vi "Run.vi"(8 "error in (no error)":errorcluster, 11 "Channel in":refnum<class "ECHARPE_Channel.lvclass">) -> (0 "error out":errorcluster, 3 "Channel out":refnum<class "ECHARPE_Channel.lvclass">)   [LabVIEW 2018, in "ECHARPE_Channel.lvclass"]
doc: "Run the channel"
uses:
  ECHARPE_Channel.lvclass
  C:/Users/Denis/Desktop/S4ACS/S4ACS/Channel/Channel.lvclass
  Channel/Channel.lvclass/Channel.ctl
  Sim_CCD/Sim_CCD.lvclass
  State Machine/State Machine.lvclass
  RxTx/RxTx.lvclass
  Server/Server.lvclass
  Channel/Channel.lvclass
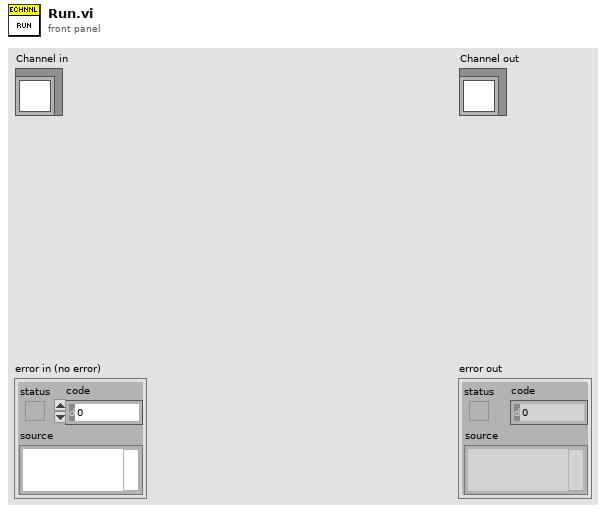
[diagram p1: front panel]
types:
  T1 = cluster{"State Machine.lvclass":refnum<class "State Machine.lvclass">, "RxTx.lvclass":refnum<class "RxTx.lvclass">, "Save_Header_RxTx.lvclass":refnum<class "RxTx.lvclass">, "Status SM.lvclass":refnum<class "State Machine.lvclass">, "Status RxTx.lvclass":refnum<class "RxTx.lvclass">, "servers array":refnum<class "Server.lvclass">[], "Events log file.lvclass":refnum<class "Log File.lvclass">, "Errors log file.lvclass":refnum<class "Log File.lvclass">, "Keywords log file.lvclass":refnum<class "Log File.lvclass">, "Sim_CCD.lvclass":refnum<class "Sim_CCD.lvclass">}
  T2 = cluster{"field 1":string, "field 2":string, "field 3":string}
  T3 = cluster{"PREAMP":u16, "READOUT_RATE":u16, "VERTICAL_SHIFT_SPEED":u16, "READ_MODE":u16, "VERTICAL_CLOCK_VOLTAGE":u16, "ACQUISITION_MODE":u16, "AD_CHANNEL":u16, "SHUTTER_TTL":u16, "SHUTTER_OPENING_TIME":u16, "SHUTTER_CLOSING_TIME":u16, "SHUTTER_MODE":u16, "TRIGGER_MODE":u16, "VBIN":u16, "INITIAL_LINE":u16, "INITIAL_COLUMN":u16, "FINAL_LINE":u16, "FINAL_COLUMN":u16, "HBIN":u16}
  T4 = typedef "LVDateTimeRec.ctl" = cluster{"fractional second":dbl, "second":i32, "minute":i32, "hour":i32, "day of month":i32, "month":i32, "year":i32, "day of week":i32, "day of year":i32, "DST":i32}
  T5 = cluster{"Time Acq Started":u32, "Image delay":u64, "Last update - CCD config":timestamp, "SYSTEMTIME":T4, "Readout time":dbl, "Time acq finished":u32, "effective exptime":dbl}
  T6 = cluster{"FRAMES_DONE":u16, "CCD_STATUS":string, "CURRENT_TEMPERATURE":i16, "TEMPERATURE_STATUS":string, "FRAME_EXPOSURE_TIME":dbl, "SERIAL_NUMBER":u16, "ACQUIRING":bool, "POWER":bool, "ACS MODE":bool}
  T7 = cluster{"Stop Acquisition":bool, "Abort Acquisition":bool, "Pause acquisition":bool, "wait expose command":bool, "video mode":bool, "stop app":bool}
  T8 = cluster{"CYCLES_DONE":u16, "LAST_IMAGE_NAME":string, "USED_DISK_SPACE":u16, "IMAGE_INDEX":u32, "acquisition error":bool}
  T9 = cluster{"EXPTIME":dbl, "#FRAMES":u32, "COOLER_POWER_STATUS":u16, "TEMP":i32}
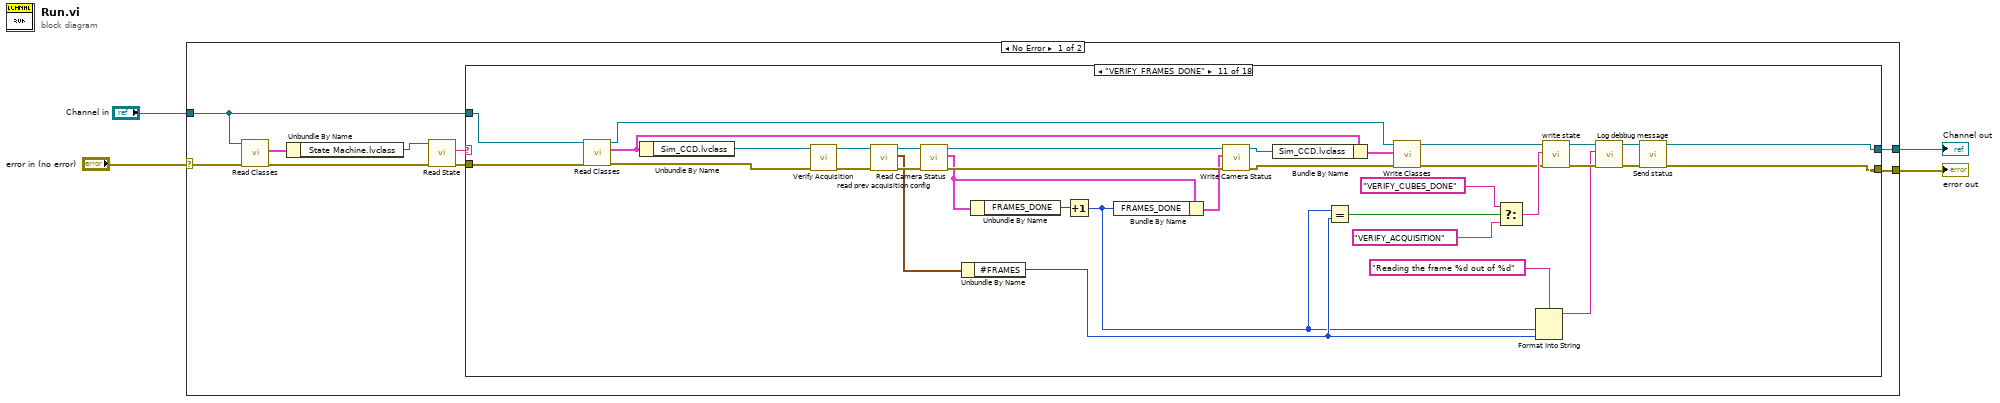
[diagram p0: block diagram]
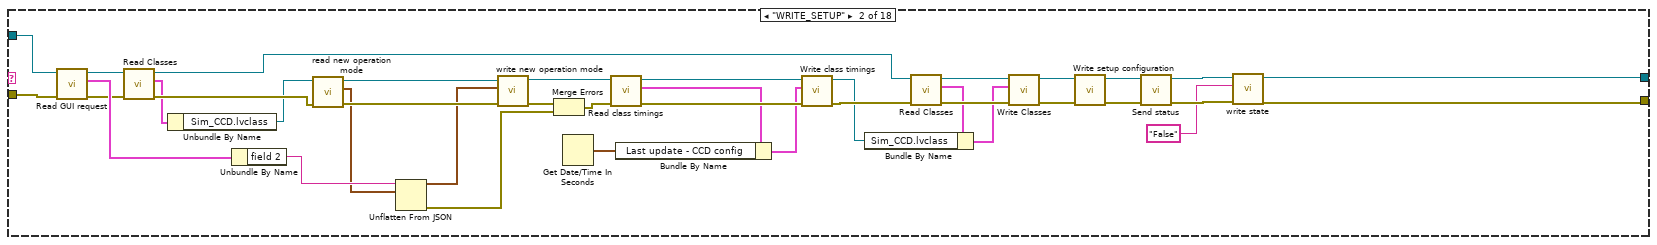
[diagram p3: hidden frame]
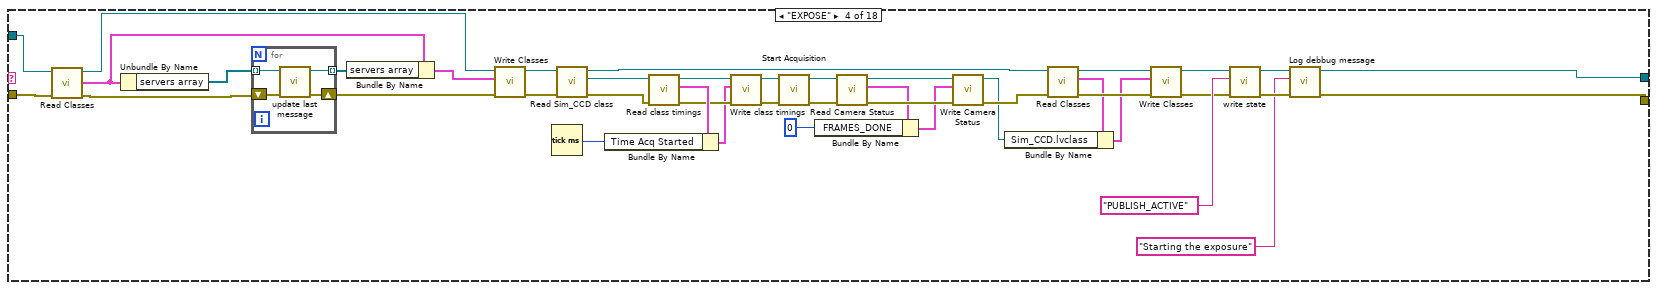
[diagram p5: hidden frame]
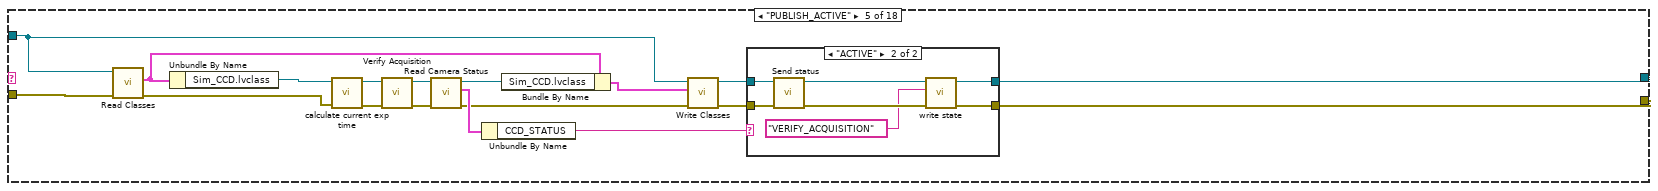
[diagram p6: hidden frame]
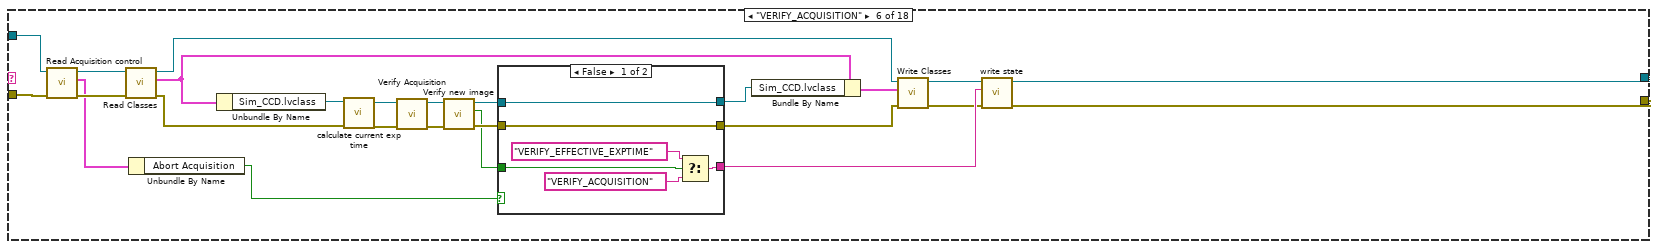
[diagram p8: hidden frame]
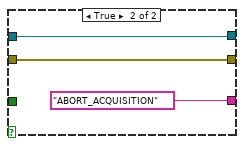
[diagram p9: hidden frame]
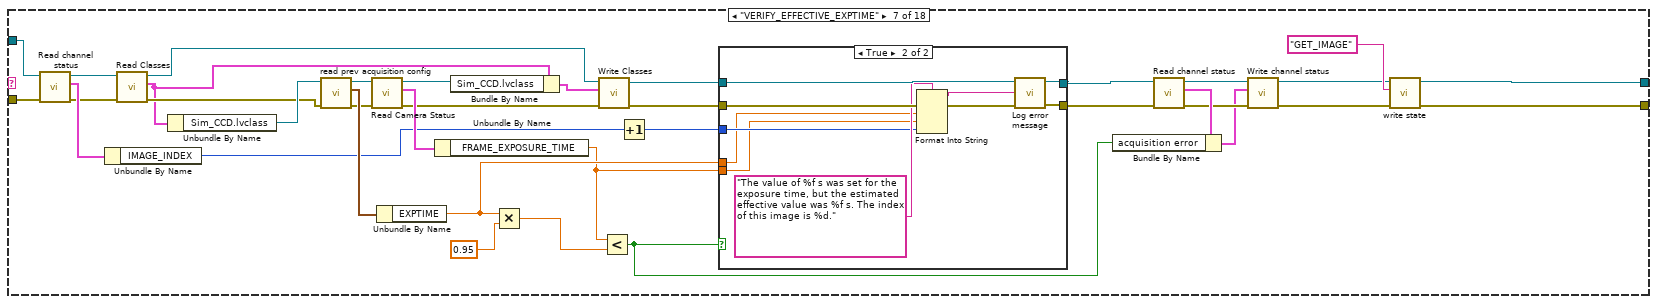
[diagram p10: hidden frame]
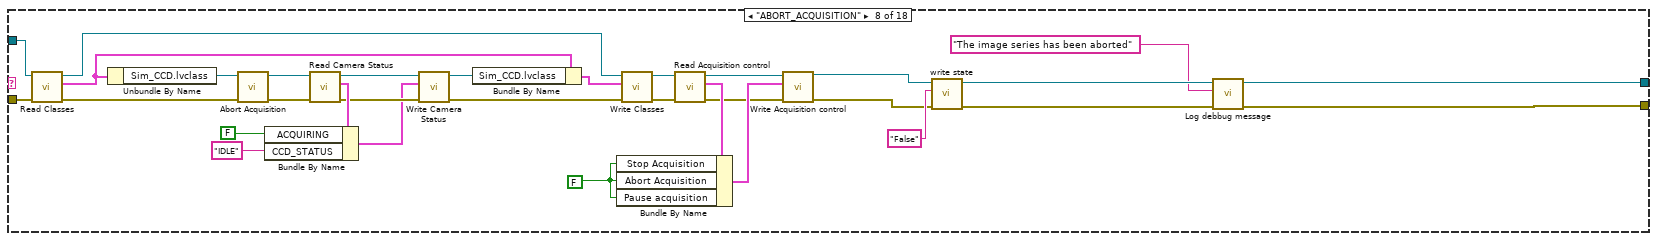
[diagram p12: hidden frame]
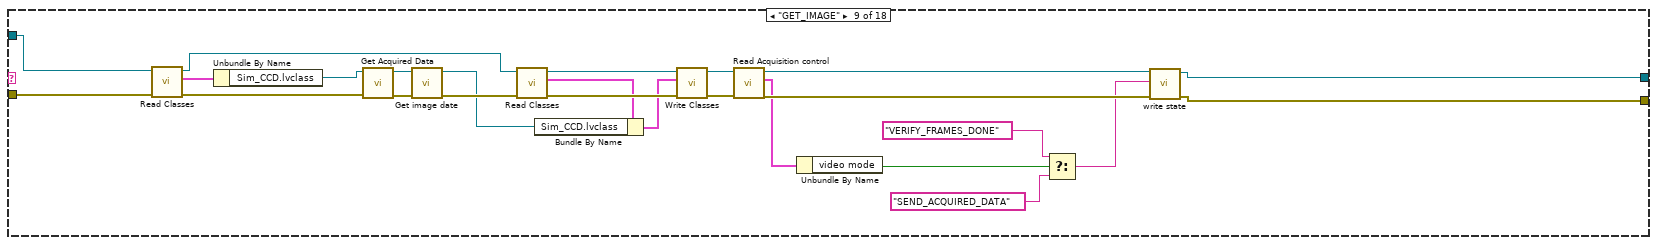
[diagram p13: hidden frame]
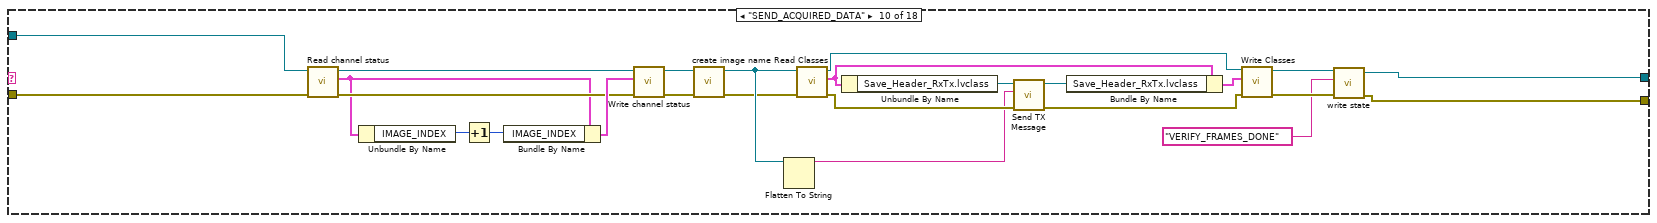
[diagram p14: hidden frame]
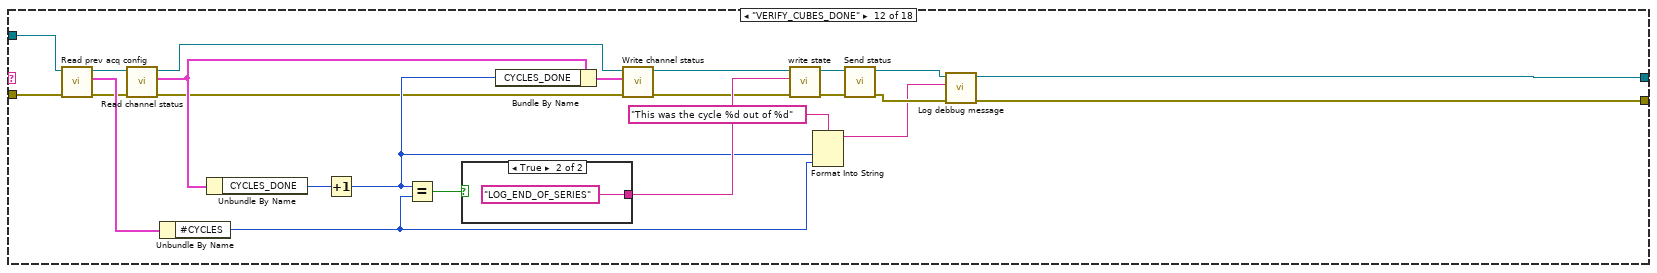
[diagram p15: hidden frame]
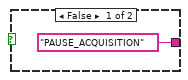
[diagram p16: hidden frame]
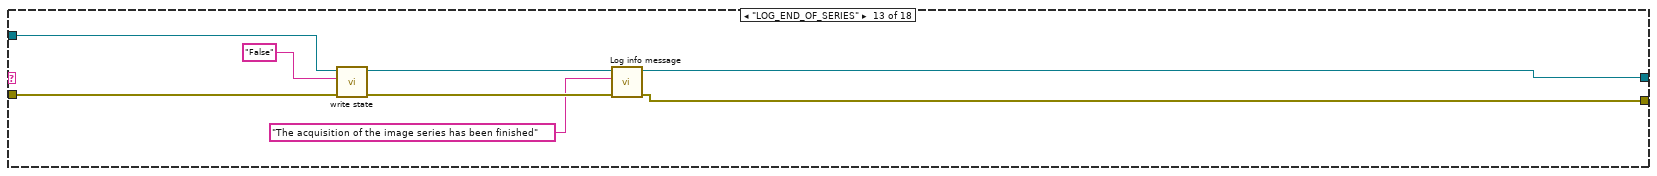
[diagram p17: hidden frame]
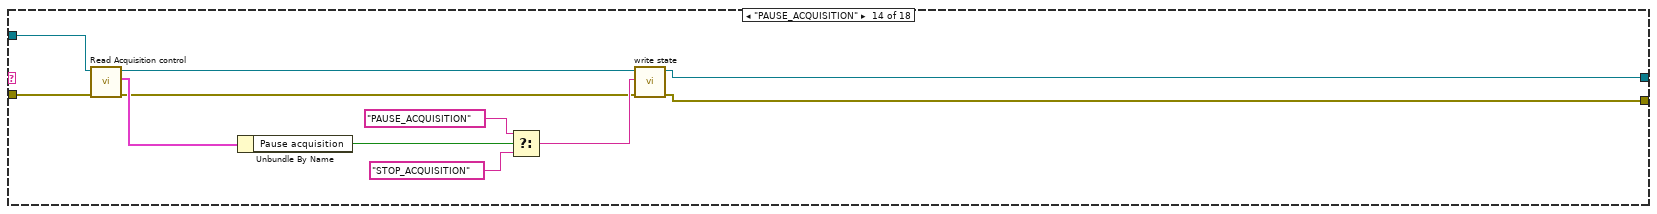
[diagram p18: hidden frame]
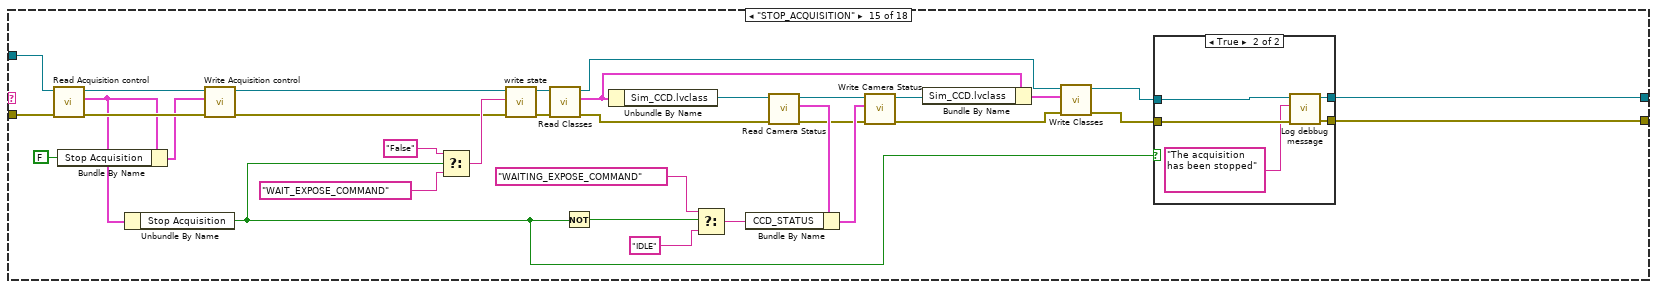
[diagram p19: hidden frame]
diagram:
  n1 = case shown="No Error" "error in (no error)" {
    selector: "error in (no error)" -> [w7 w552]
    tunnel: [w13 w552] -> w3
    tunnel: [w12 w551] -> w1
    tunnel: "Channel in" -> [w8 w551]
    frame No Error {
      n2 = call-dynamic "Read Classes.vi"("error in (no error)"=w7, "Channel in"=w8) -> ("error out"=w6:errorcluster, "Classes"=w9:T1)  [unwired: 7 in, 1 out]
      n3 = Unbundle By Name(w9) -> ("State Machine.lvclass"=w5:refnum<class "State Machine.lvclass">)
      n4 = call-dynamic "Read State.vi"("error in (no error)"=w6, "State Machine in"=w5) -> ("error out"=w11:errorcluster, "State"=w10:string)  [unwired: 7 in, 1 out]
      n5 = case shown="\"VERIFY_FRAMES_DONE\"" w10 {
        tunnel: w11 -> [w14 w36 w54 w77 w111 w134 w175 w228 w262 w271 w317 w334 w360 w364 w391 w416 w425 w432]
        tunnel: [w14 w23 w54 w87 w118 w150 w197 w231 w253 w291 w316 w346 w356 w370 w394 w422 w425 w442] -> w13
        tunnel: [w15 w24 w55 w88 w119 w151 w198 w232 w252 w292 w315 w345 w357 w369 w395 w421 w426 w443] -> w12
        tunnel: w8 -> [w15 w38 w55 w76 w106 w132 w169 w227 w263 w272 w318 w332 w361 w365 w392 w417 w426 w431]
        frame "False", Default {
        }
        frame "WRITE_SETUP" {
          n6 = call "Read GUI request.vi"("error in (no error)"=w36, "Channel in"=w38) -> ("error out"=w37:errorcluster, "GUI request"=w42:T2, "Channel out"=w39:refnum<class "ECHARPE_Channel.lvclass">)  [unwired: 7 in]
          n7 = call-dynamic "Read Classes.vi"("error in (no error)"=w37, "Channel in"=w39) -> ("error out"=w40:errorcluster, "Classes"=w17:T1, "Channel out"=w29:refnum<class "ECHARPE_Channel.lvclass">)  [unwired: 7 in]
          n8 = Unbundle By Name(w17) -> ("Sim_CCD.lvclass"=w16:refnum<class "Sim_CCD.lvclass">)
          n9 = Unbundle By Name(w42) -> ("field 2"=w41:string)
          n10 = call "read new operation mode.vi"("error in (no error)"=w40, "CCDCamera in"=w16) -> ("error out"=w52:errorcluster, "new operation mode"=w19:T3, "CCDCamera out"=w53:refnum<class "Sim_CCD.lvclass">)  [unwired: 7 in]
          n11 = Unflatten From JSON(JSON string=w41, type and defaults=w19) -> (value=w18:T3, error out=w43:errorcluster)  [unwired: 5 in]
          n12 = call "write new operation mode.vi"("error in (no error)"=w52, "new operation mode"=w18, "CCDCamera in"=w53) -> ("error out"=w45:errorcluster, "CCDCamera out"=w51:refnum<class "Sim_CCD.lvclass">)  [unwired: 7 in]
          n13 = Merge Errors(w45, w43) -> (w44:errorcluster)
          n14 = Get Date/Time In Seconds() -> (seconds since 1Jan1904=w46:timestamp)
          n15 = call "Read class timings.vi"("error in (no error)"=w44, "Simulated Camera in"=w51) -> ("error out"=w49:errorcluster, "class timings"=w48:T5, "Simulated Camera out"=w50:refnum<class "Sim_CCD.lvclass">)  [unwired: 7 in]
          n16 = Bundle By Name(cluster=w48, "Last update - CCD config"=w46) -> (w47:T5)
          n17 = call "Write class timings.vi"("error in (no error)"=w49, "class timings"=w47, "Simulated Camera in"=w50) -> ("error out"=w33:errorcluster, "Simulated Camera out"=w31:refnum<class "Sim_CCD.lvclass">)  [unwired: 7 in]
          n18 = call-dynamic "Read Classes.vi"("error in (no error)"=w33, "Channel in"=w29) -> ("error out"=w34:errorcluster, "Classes"=w32:T1, "Channel out"=w35:refnum<class "ECHARPE_Channel.lvclass">)  [unwired: 7 in]
          n19 = Bundle By Name(cluster=w32, "Sim_CCD.lvclass"=w31) -> (w30:T1)
          n20 = call-dynamic "Write Classes.vi"("error in (no error)"=w34, "Classes"=w30, "Channel in"=w35) -> ("error out"=w25:errorcluster, "Channel out"=w27:refnum<class "ECHARPE_Channel.lvclass">)  [unwired: 7 in]
          n21 = call "Write setup configuration.vi"("error in (no error)"=w25, "Channel in"=w27) -> ("error out"=w26:errorcluster, "Channel out"=w28:refnum<class "ECHARPE_Channel.lvclass">)  [unwired: 8 in]
          n22 = call-dynamic "Send status.vi"("error in (no error)"=w26, "Channel in"=w28) -> ("error out"=w21:errorcluster, "Channel out"=w22:refnum<class "ECHARPE_Channel.lvclass">)  [unwired: 8 in]
          n23 = call "write state.vi"("error in (no error)"=w21, "state"="False", "Channel in"=w22) -> ("error out"=w23:errorcluster, "Channel out"=w24:refnum<class "ECHARPE_Channel.lvclass">)  [unwired: 7 in]
        }
        frame "---------------------------------" {
        }
        frame "EXPOSE" {
          n24 = call-dynamic "Read Classes.vi"("error in (no error)"=w77, "Channel in"=w76) -> ("error out"=w73:errorcluster, "Classes"=w70:T1, "Channel out"=w74:refnum<class "ECHARPE_Channel.lvclass">)  [unwired: 7 in]
          n25 = Unbundle By Name(w70) -> ("servers array"=w75:refnum<class "Server.lvclass">[])
          n26 = for {
            tunnel: w75 -> [w98] mode=indexing
            shift-right: [w101] -> w72
            shift-left: w73 -> [w99]
            tunnel: [w100] -> w69 mode=indexing
            n27 = call "update last message.vi"("error in (no error)"=w99, "Server in"=w98) -> ("error out"=w101:errorcluster, "Server out"=w100:refnum<class "Server.lvclass">)  [unwired: 8 in]
          }
          n28 = Bundle By Name(cluster=w70, "servers array"=w69) -> (w71:T1)
          n29 = call-dynamic "Write Classes.vi"("error in (no error)"=w72, "Classes"=w71, "Channel in"=w74) -> ("error out"=w66:errorcluster, "Channel out"=w67:refnum<class "ECHARPE_Channel.lvclass">)  [unwired: 7 in]
          n30 = Tick Count (ms)() -> (millisecond timer value=w78:u32)
          n31 = call "Read Sim_CCD class.vi"("error in (no error)"=w66, "Channel in"=w67) -> ("error out"=w65:errorcluster, "Sim_CCD.lvclass"=w68:refnum<class "Sim_CCD.lvclass">, "Channel out"=w59:refnum<class "ECHARPE_Channel.lvclass">)  [unwired: 7 in]
          n32 = call "Read class timings.vi"("error in (no error)"=w65, "Simulated Camera in"=w68) -> ("error out"=w81:errorcluster, "class timings"=w82:T5, "Simulated Camera out"=w80:refnum<class "Sim_CCD.lvclass">)  [unwired: 7 in]
          n33 = Bundle By Name(cluster=w82, "Time Acq Started"=w78) -> (w79:T5)
          n34 = call "Write class timings.vi"("error in (no error)"=w81, "class timings"=w79, "Simulated Camera in"=w80) -> ("error out"=w84:errorcluster, "Simulated Camera out"=w83:refnum<class "Sim_CCD.lvclass">)  [unwired: 7 in]
          n35 = call-dynamic "Start Acquisition.vi"("error in (no error)"=w84, "CCDCamera in"=w83) -> ("error out"=w90:errorcluster, "CCDCamera out"=w91:refnum<class "Sim_CCD.lvclass">)  [unwired: 8 in]
          n36 = call "Read Camera Status.vi"("error in (no error)"=w90, "CCDCamera in"=w91) -> ("error out"=w97:errorcluster, "camera status"=w95:T6, "CCDCamera out"=w96:refnum<class "Sim_CCD.lvclass">)  [unwired: 7 in]
          n37 = Bundle By Name(cluster=w95, "FRAMES_DONE"=u16 0) -> (w94:T6)
          n38 = call "Write Camera Status.vi"("error in (no error)"=w97, "camera status"=w94, "CCDCamera in"=w96) -> ("error out"=w64:errorcluster, "CCDCamera out"=w56:refnum<class "Sim_CCD.lvclass">)  [unwired: 7 in]
          n39 = call-dynamic "Read Classes.vi"("error in (no error)"=w64, "Channel in"=w59) -> ("error out"=w61:errorcluster, "Classes"=w58:T1, "Channel out"=w60:refnum<class "ECHARPE_Channel.lvclass">)  [unwired: 7 in]
          n40 = Bundle By Name(cluster=w58, "Sim_CCD.lvclass"=w56) -> (w57:T1)
          n41 = call-dynamic "Write Classes.vi"("error in (no error)"=w61, "Classes"=w57, "Channel in"=w60) -> ("error out"=w63:errorcluster, "Channel out"=w62:refnum<class "ECHARPE_Channel.lvclass">)  [unwired: 7 in]
          n42 = call "write state.vi"("error in (no error)"=w63, "state"="PUBLISH_ACTIVE", "Channel in"=w62) -> ("error out"=w86:errorcluster, "Channel out"=w89:refnum<class "ECHARPE_Channel.lvclass">)  [unwired: 7 in]
          n43 = call "Log debbug message.vi"("error in (no error)"=w86, "String"="Starting the exposure", "Channel in"=w89) -> ("error out"=w87:errorcluster, "Channel out"=w88:refnum<class "ECHARPE_Channel.lvclass">)  [unwired: 7 in]
        }
        frame "PUBLISH_ACTIVE" {
          n44 = call-dynamic "Read Classes.vi"("error in (no error)"=w111, "Channel in"=w106) -> ("error out"=w109:errorcluster, "Classes"=w104:T1)  [unwired: 7 in, 1 out]
          n45 = Unbundle By Name(w104) -> ("Sim_CCD.lvclass"=w110:refnum<class "Sim_CCD.lvclass">)
          n46 = call-dynamic "calculate current exp time.vi"("error in (no error)"=w109, "CCDCamera in"=w110) -> ("error out"=w112:errorcluster, "CCDCamera out"=w113:refnum<class "Sim_CCD.lvclass">)  [unwired: 8 in]
          n47 = call-dynamic "Verify Acquisition.vi"("error in (no error)"=w112, "CCDCamera in"=w113) -> ("error out"=w114:errorcluster, "CCDCamera out"=w115:refnum<class "Sim_CCD.lvclass">)  [unwired: 8 in]
          n48 = call "Read Camera Status.vi"("error in (no error)"=w114, "CCDCamera in"=w115) -> ("error out"=w105:errorcluster, "camera status"=w117:T6, "CCDCamera out"=w103:refnum<class "Sim_CCD.lvclass">)  [unwired: 7 in]
          n49 = Unbundle By Name(w117) -> ("CCD_STATUS"=w116:string)
          n50 = Bundle By Name(cluster=w104, "Sim_CCD.lvclass"=w103) -> (w102:T1)
          n51 = call-dynamic "Write Classes.vi"("error in (no error)"=w105, "Classes"=w102, "Channel in"=w106) -> ("error out"=w107:errorcluster, "Channel out"=w108:refnum<class "ECHARPE_Channel.lvclass">)  [unwired: 7 in]
          n52 = case shown="\"ACTIVE\"" w116 {
            tunnel: w108 -> [w121 w124]
            tunnel: [w121 w128] -> w119
            tunnel: [w120 w127] -> w118
            tunnel: w107 -> [w120 w123]
            frame "False", Default {
            }
            frame "ACTIVE" {
              n53 = call-dynamic "Send status.vi"("error in (no error)"=w123, "Channel in"=w124) -> ("error out"=w126:errorcluster, "Channel out"=w125:refnum<class "ECHARPE_Channel.lvclass">)  [unwired: 8 in]
              n54 = call "write state.vi"("error in (no error)"=w126, "state"="VERIFY_ACQUISITION", "Channel in"=w125) -> ("error out"=w127:errorcluster, "Channel out"=w128:refnum<class "ECHARPE_Channel.lvclass">)  [unwired: 7 in]
            }
          }
        }
        frame "VERIFY_ACQUISITION" {
          n55 = call "Read Acquisition control.vi"("error in (no error)"=w134, "Channel in"=w132) -> ("error out"=w133:errorcluster, "Acquisition control"=w130:T7, "Channel out"=w131:refnum<class "ECHARPE_Channel.lvclass">)  [unwired: 7 in]
          n56 = call-dynamic "Read Classes.vi"("error in (no error)"=w133, "Channel in"=w131) -> ("error out"=w140:errorcluster, "Classes"=w137:T1, "Channel out"=w139:refnum<class "ECHARPE_Channel.lvclass">)  [unwired: 7 in]
          n57 = Unbundle By Name(w130) -> ("Abort Acquisition"=w129:bool)
          n58 = Unbundle By Name(w137) -> ("Sim_CCD.lvclass"=w138:refnum<class "Sim_CCD.lvclass">)
          n59 = call-dynamic "calculate current exp time.vi"("error in (no error)"=w140, "CCDCamera in"=w138) -> ("error out"=w146:errorcluster, "CCDCamera out"=w147:refnum<class "Sim_CCD.lvclass">)  [unwired: 8 in]
          n60 = call-dynamic "Verify Acquisition.vi"("error in (no error)"=w146, "CCDCamera in"=w147) -> ("error out"=w153:errorcluster, "CCDCamera out"=w152:refnum<class "Sim_CCD.lvclass">)  [unwired: 8 in]
          n61 = call-dynamic "Verify new image.vi"("error in (no error)"=w153, "CCDCamera in"=w152) -> ("error out"=w148:errorcluster, "New Images ?"=w144:bool, "CCDCamera out"=w149:refnum<class "Sim_CCD.lvclass">)  [unwired: 7 in]
          n62 = case shown="False" w129 {
            tunnel: w149 -> [w159 w162]
            tunnel: w148 -> [w158 w161]
            tunnel: [w159 w162] -> w135
            tunnel: [w158 w161] -> w141
            tunnel: [w155 "ABORT_ACQUISITION"] -> w145
            tunnel: w144 -> [w154 _]
            frame False {
              n63 = Select(t="VERIFY_EFFECTIVE_EXPTIME", s=w154, f="VERIFY_ACQUISITION") -> (s? t:f=w155:string)
            }
            frame True {
            }
          }
          n64 = Bundle By Name(cluster=w137, "Sim_CCD.lvclass"=w135) -> (w136:T1)
          n65 = call-dynamic "Write Classes.vi"("error in (no error)"=w141, "Classes"=w136, "Channel in"=w139) -> ("error out"=w143:errorcluster, "Channel out"=w142:refnum<class "ECHARPE_Channel.lvclass">)  [unwired: 7 in]
          n66 = call "write state.vi"("error in (no error)"=w143, "state"=w145, "Channel in"=w142) -> ("error out"=w150:errorcluster, "Channel out"=w151:refnum<class "ECHARPE_Channel.lvclass">)  [unwired: 7 in]
        }
        frame "VERIFY_EFFECTIVE_EXPTIME" {
          n67 = call-dynamic "Read channel status.vi"("error in (no error)"=w175, "Channel in"=w169) -> ("error out"=w174:errorcluster, "channel status"=w177:T8, "Channel out"=w173:refnum<class "ECHARPE_Channel.lvclass">)  [unwired: 7 in]
          n68 = Unbundle By Name(w177) -> ("IMAGE_INDEX"=w176:u32)
          n69 = call-dynamic "Read Classes.vi"("error in (no error)"=w174, "Channel in"=w173) -> ("error out"=w171:errorcluster, "Classes"=w165:T1, "Channel out"=w168:refnum<class "ECHARPE_Channel.lvclass">)  [unwired: 7 in]
          n70 = Unbundle By Name(w165) -> ("Sim_CCD.lvclass"=w172:refnum<class "Sim_CCD.lvclass">)
          n71 = call "read prev acquisition config.vi"("error in (no error)"=w171, "Simulated_CCD_Camera in"=w172) -> ("error out"=w191:errorcluster, "prev acquisition configuration"=w193:T9, "Simulated_CCD_Camera out"=w192:refnum<class "Sim_CCD.lvclass">)  [unwired: 7 in]
          n72 = call "Read Camera Status.vi"("error in (no error)"=w191, "CCDCamera in"=w192) -> ("error out"=w166:errorcluster, "camera status"=w190:T6, "CCDCamera out"=w163:refnum<class "Sim_CCD.lvclass">)  [unwired: 7 in]
          n73 = Unbundle By Name(w193) -> ("EXPTIME"=w188:dbl)
          n74 = Unbundle By Name(w190) -> ("FRAME_EXPOSURE_TIME"=w187:dbl)
          n75 = Bundle By Name(cluster=w165, "Sim_CCD.lvclass"=w163) -> (w164:T1)
          n76 = Multiply(x=w188, y=0.95) -> (x*y=w194:dbl)
          n77 = call-dynamic "Write Classes.vi"("error in (no error)"=w166, "Classes"=w164, "Channel in"=w168) -> ("error out"=w170:errorcluster, "Channel out"=w167:refnum<class "ECHARPE_Channel.lvclass">)  [unwired: 7 in]
          n78 = Less?(x=w187, y=w194) -> (x < y?=w185:bool)
          n79 = Increment(x=w176) -> (x+1=w189:u32)
          n80 = case shown="True" w185 {
            tunnel: w167 -> [w200 w210]
            tunnel: [w200 w209] -> w184
            tunnel: [w199 w208] -> w183
            tunnel: w170 -> [w199 w207]
            tunnel: w189 -> [_ w203]
            tunnel: w188 -> [_ w202]
            tunnel: w187 -> [_ w201]
            frame False {
            }
            frame True {
              n81 = Format Into String(format string="The value of %f s was set for the exposure time, but the estimated effective value was %f s. The index of this image is %d.", error in=w207, w202, w201, w203) -> (resulting string=w204:string, error out=w206:errorcluster)  [unwired: 1 in]
              n82 = call "Log error message.vi"("error in (no error)"=w206, "String"=w204, "Channel in"=w210) -> ("error out"=w208:errorcluster, "Channel out"=w209:refnum<class "ECHARPE_Channel.lvclass">)  [unwired: 7 in]
            }
          }
          n83 = call-dynamic "Read channel status.vi"("error in (no error)"=w183, "Channel in"=w184) -> ("error out"=w179:errorcluster, "channel status"=w186:T8, "Channel out"=w180:refnum<class "ECHARPE_Channel.lvclass">)  [unwired: 7 in]
          n84 = Bundle By Name(cluster=w186, "acquisition error"=w185) -> (w178:T8)
          n85 = call-dynamic "Write channel status.vi"("error in (no error)"=w179, "channel status"=w178, "Channel in"=w180) -> ("error out"=w182:errorcluster, "Channel out"=w181:refnum<class "ECHARPE_Channel.lvclass">)  [unwired: 7 in]
          n86 = call "write state.vi"("error in (no error)"=w182, "state"="GET_IMAGE", "Channel in"=w181) -> ("error out"=w197:errorcluster, "Channel out"=w198:refnum<class "ECHARPE_Channel.lvclass">)  [unwired: 7 in]
        }
        frame "ABORT_ACQUISITION" {
          w211 = FALSE ("Acquiring")
          n87 = call-dynamic "Read Classes.vi"("error in (no error)"=w228, "Channel in"=w227) -> ("error out"=w225:errorcluster, "Classes"=w221:T1, "Channel out"=w220:refnum<class "ECHARPE_Channel.lvclass">)  [unwired: 7 in]
          n88 = Unbundle By Name(w221) -> ("Sim_CCD.lvclass"=w226:refnum<class "Sim_CCD.lvclass">)
          n89 = call-dynamic "Abort Acquisition.vi"("error in (no error)"=w225, "CCDCamera in"=w226) -> ("error out"=w239:errorcluster, "CCDCamera out"=w240:refnum<class "Sim_CCD.lvclass">)  [unwired: 8 in]
          n90 = call "Read Camera Status.vi"("error in (no error)"=w239, "CCDCamera in"=w240) -> ("error out"=w237:errorcluster, "camera status"=w242:T6, "CCDCamera out"=w238:refnum<class "Sim_CCD.lvclass">)  [unwired: 7 in]
          n91 = Bundle By Name(cluster=w242, "ACQUIRING"=FALSE ("Acquiring"), "CCD_STATUS"="IDLE" ("STATUS")) -> (w236:T6)
          n92 = call "Write Camera Status.vi"("error in (no error)"=w237, "camera status"=w236, "CCDCamera in"=w238) -> ("error out"=w223:errorcluster, "CCDCamera out"=w224:refnum<class "Sim_CCD.lvclass">)  [unwired: 7 in]
          n93 = Bundle By Name(cluster=w221, "Sim_CCD.lvclass"=w224) -> (w222:T1)
          n94 = call-dynamic "Write Classes.vi"("error in (no error)"=w223, "Classes"=w222, "Channel in"=w220) -> ("error out"=w218:errorcluster, "Channel out"=w219:refnum<class "ECHARPE_Channel.lvclass">)  [unwired: 7 in]
          n95 = call "Read Acquisition control.vi"("error in (no error)"=w218, "Channel in"=w219) -> ("error out"=w212:errorcluster, "Acquisition control"=w214:T7, "Channel out"=w217:refnum<class "ECHARPE_Channel.lvclass">)  [unwired: 7 in]
          n96 = Bundle By Name(cluster=w214, "Stop Acquisition"=w211, "Abort Acquisition"=w211, "Pause acquisition"=w211) -> (w213:T7)
          n97 = call "Write Acquisition control.vi"("error in (no error)"=w212, "Acquisition control"=w213, "Channel in"=w217) -> ("error out"=w215:errorcluster, "Channel out"=w216:refnum<class "ECHARPE_Channel.lvclass">)  [unwired: 7 in]
          n98 = call "write state.vi"("error in (no error)"=w215, "state"="False", "Channel in"=w216) -> ("error out"=w230:errorcluster, "Channel out"=w233:refnum<class "ECHARPE_Channel.lvclass">)  [unwired: 7 in]
          n99 = call "Log debbug message.vi"("error in (no error)"=w230, "String"="The image series has been aborted", "Channel in"=w233) -> ("error out"=w231:errorcluster, "Channel out"=w232:refnum<class "ECHARPE_Channel.lvclass">)  [unwired: 7 in]
        }
        frame "GET_IMAGE" {
          n100 = call-dynamic "Read Classes.vi"("error in (no error)"=w262, "Channel in"=w263) -> ("error out"=w260:errorcluster, "Classes"=w261:T1, "Channel out"=w258:refnum<class "ECHARPE_Channel.lvclass">)  [unwired: 7 in]
          n101 = Unbundle By Name(w261) -> ("Sim_CCD.lvclass"=w259:refnum<class "Sim_CCD.lvclass">)
          n102 = call-dynamic "Get Acquired Data.vi"("error in (no error)"=w260, "CCDCamera in"=w259) -> ("error out"=w266:errorcluster, "CCDCamera out"=w267:refnum<class "Sim_CCD.lvclass">)  [unwired: 8 in]
          n103 = call-dynamic "Get image date.vi"("error in (no error)"=w266, "Simulated_CCD_Camera in"=w267) -> ("error out"=w265:errorcluster, "Simulated_CCD_Camera out"=w264:refnum<class "Sim_CCD.lvclass">)  [unwired: 8 in]
          n104 = call-dynamic "Read Classes.vi"("error in (no error)"=w265, "Channel in"=w258) -> ("error out"=w257:errorcluster, "Classes"=w256:T1, "Channel out"=w255:refnum<class "ECHARPE_Channel.lvclass">)  [unwired: 7 in]
          n105 = Bundle By Name(cluster=w256, "Sim_CCD.lvclass"=w264) -> (w254:T1)
          n106 = call-dynamic "Write Classes.vi"("error in (no error)"=w257, "Classes"=w254, "Channel in"=w255) -> ("error out"=w250:errorcluster, "Channel out"=w251:refnum<class "ECHARPE_Channel.lvclass">)  [unwired: 7 in]
          n107 = call "Read Acquisition control.vi"("error in (no error)"=w250, "Channel in"=w251) -> ("error out"=w248:errorcluster, "Acquisition control"=w247:T7, "Channel out"=w249:refnum<class "ECHARPE_Channel.lvclass">)  [unwired: 7 in]
          n108 = Unbundle By Name(w247) -> ("video mode"=w246:bool)
          n109 = Select(t="VERIFY_FRAMES_DONE", s=w246, f="SEND_ACQUIRED_DATA") -> (s? t:f=w243:string)
          n110 = call "write state.vi"("error in (no error)"=w248, "state"=w243, "Channel in"=w249) -> ("error out"=w253:errorcluster, "Channel out"=w252:refnum<class "ECHARPE_Channel.lvclass">)  [unwired: 7 in]
        }
        frame "SEND_ACQUIRED_DATA" {
          n111 = call-dynamic "Read channel status.vi"("error in (no error)"=w271, "Channel in"=w272) -> ("error out"=w278:errorcluster, "channel status"=w270:T8, "Channel out"=w277:refnum<class "ECHARPE_Channel.lvclass">)  [unwired: 7 in]
          n112 = Unbundle By Name(w270) -> ("IMAGE_INDEX"=w269:u32)
          n113 = Increment(x=w269) -> (x+1=w268:u32)
          n114 = Bundle By Name(cluster=w270, "IMAGE_INDEX"=w268) -> (w279:T8)
          n115 = call-dynamic "Write channel status.vi"("error in (no error)"=w278, "channel status"=w279, "Channel in"=w277) -> ("error out"=w273:errorcluster, "Channel out"=w274:refnum<class "ECHARPE_Channel.lvclass">)  [unwired: 7 in]
          n116 = call-dynamic "create image name.vi"("error in (no error)"=w273, "Channel in"=w274) -> ("error out"=w275:errorcluster, "Channel out"=w276:refnum<class "ECHARPE_Channel.lvclass">)  [unwired: 8 in]
          n117 = Flatten To String(anything=w276) -> (data string=w281:string)  [unwired: 3 in, 2 out]
          n118 = call-dynamic "Read Classes.vi"("error in (no error)"=w275, "Channel in"=w276) -> ("error out"=w286:errorcluster, "Classes"=w285:T1, "Channel out"=w280:refnum<class "ECHARPE_Channel.lvclass">)  [unwired: 7 in]
          n119 = Unbundle By Name(w285) -> ("Save_Header_RxTx.lvclass"=w287:refnum<class "RxTx.lvclass">)
          n120 = call "Send TX Message.vi"("error in (no error)"=w286, "message"=w281, "RxTx in"=w287) -> ("error out"=w282:errorcluster, "RxTx out"=w283:refnum<class "RxTx.lvclass">)  [unwired: 7 in]
          n121 = Bundle By Name(cluster=w285, "Save_Header_RxTx.lvclass"=w283) -> (w284:T1)
          n122 = call-dynamic "Write Classes.vi"("error in (no error)"=w282, "Classes"=w284, "Channel in"=w280) -> ("error out"=w290:errorcluster, "Channel out"=w289:refnum<class "ECHARPE_Channel.lvclass">)  [unwired: 7 in]
          n123 = call "write state.vi"("error in (no error)"=w290, "state"="VERIFY_FRAMES_DONE", "Channel in"=w289) -> ("error out"=w291:errorcluster, "Channel out"=w292:refnum<class "ECHARPE_Channel.lvclass">)  [unwired: 7 in]
        }
        frame "VERIFY_FRAMES_DONE" {
          n124 = call-dynamic "Read Classes.vi"("error in (no error)"=w317, "Channel in"=w318) -> ("error out"=w293:errorcluster, "Classes"=w320:T1, "Channel out"=w319:refnum<class "ECHARPE_Channel.lvclass">)  [unwired: 7 in]
          n125 = Unbundle By Name(w320) -> ("Sim_CCD.lvclass"=w294:refnum<class "Sim_CCD.lvclass">)
          n126 = call-dynamic "Verify Acquisition.vi"("error in (no error)"=w293, "CCDCamera in"=w294) -> ("error out"=w295:errorcluster, "CCDCamera out"=w296:refnum<class "Sim_CCD.lvclass">)  [unwired: 8 in]
          n127 = call "read prev acquisition config.vi"("error in (no error)"=w295, "Simulated_CCD_Camera in"=w296) -> ("error out"=w305:errorcluster, "prev acquisition configuration"=w303:T9, "Simulated_CCD_Camera out"=w304:refnum<class "Sim_CCD.lvclass">)  [unwired: 7 in]
          n128 = call "Read Camera Status.vi"("error in (no error)"=w305, "CCDCamera in"=w304) -> ("error out"=w310:errorcluster, "camera status"=w306:T6, "CCDCamera out"=w309:refnum<class "Sim_CCD.lvclass">)  [unwired: 7 in]
          n129 = Unbundle By Name(w303) -> ("#FRAMES"=w298:u32)
          n130 = Unbundle By Name(w306) -> ("FRAMES_DONE"=w308:u16)
          n131 = Increment(x=w308) -> (x+1=w297:u16)
          n132 = Bundle By Name(cluster=w306, "FRAMES_DONE"=w297) -> (w307:T6)
          n133 = call "Write Camera Status.vi"("error in (no error)"=w310, "camera status"=w307, "CCDCamera in"=w309) -> ("error out"=w299:errorcluster, "CCDCamera out"=w300:refnum<class "Sim_CCD.lvclass">)  [unwired: 7 in]
          n134 = Bundle By Name(cluster=w320, "Sim_CCD.lvclass"=w300) -> (w321:T1)
          n135 = Equal?(x=w297, y=w298) -> (x = y?=w327:bool)
          n136 = call-dynamic "Write Classes.vi"("error in (no error)"=w299, "Classes"=w321, "Channel in"=w319) -> ("error out"=w322:errorcluster, "Channel out"=w323:refnum<class "ECHARPE_Channel.lvclass">)  [unwired: 7 in]
          n137 = Select(t="VERIFY_CUBES_DONE", s=w327, f="VERIFY_ACQUISITION") -> (s? t:f=w324:string)
          n138 = Format Into String(format string="Reading the frame %d out of %d", w297, w298) -> (resulting string=w301:string)  [unwired: 2 in, 1 out]
          n139 = call "write state.vi"("error in (no error)"=w322, "state"=w324, "Channel in"=w323) -> ("error out"=w311:errorcluster, "Channel out"=w314:refnum<class "ECHARPE_Channel.lvclass">)  [unwired: 7 in]
          n140 = call "Log debbug message.vi"("error in (no error)"=w311, "String"=w301, "Channel in"=w314) -> ("error out"=w312:errorcluster, "Channel out"=w313:refnum<class "ECHARPE_Channel.lvclass">)  [unwired: 7 in]
          n141 = call-dynamic "Send status.vi"("error in (no error)"=w312, "Channel in"=w313) -> ("error out"=w316:errorcluster, "Channel out"=w315:refnum<class "ECHARPE_Channel.lvclass">)  [unwired: 8 in]
        }
        frame "VERIFY_CUBES_DONE" {
          n142 = call-dynamic "Read prev acq config.vi"("error in (no error)"=w334, "Channel in"=w332) -> ("error out"=w333:errorcluster, "prev acq config"=w340:cluster{"suffix":string, "#CYCLES":u32}, "Channel out"=w331:refnum<class "ECHARPE_Channel.lvclass">)  [unwired: 7 in]
          n143 = call-dynamic "Read channel status.vi"("error in (no error)"=w333, "Channel in"=w331) -> ("error out"=w330:errorcluster, "channel status"=w337:T8, "Channel out"=w329:refnum<class "ECHARPE_Channel.lvclass">)  [unwired: 7 in]
          n144 = Unbundle By Name(w340) -> ("#CYCLES"=w339:u32)
          n145 = Unbundle By Name(w337) -> ("CYCLES_DONE"=w341:u16)
          n146 = Increment(x=w341) -> (x+1=w336:u16)
          n147 = Equal?(x=w336, y=w339) -> (x = y?=w351:bool)
          n148 = case shown="True" w351 {
            tunnel: ["PAUSE_ACQUISITION" "LOG_END_OF_SERIES"] -> w348
            frame False {
            }
            frame True {
            }
          }
          n149 = Bundle By Name(cluster=w337, "CYCLES_DONE"=w336) -> (w335:T8)
          n150 = call-dynamic "Write channel status.vi"("error in (no error)"=w330, "channel status"=w335, "Channel in"=w329) -> ("error out"=w338:errorcluster, "Channel out"=w328:refnum<class "ECHARPE_Channel.lvclass">)  [unwired: 7 in]
          n151 = call "write state.vi"("error in (no error)"=w338, "state"=w348, "Channel in"=w328) -> ("error out"=w349:errorcluster, "Channel out"=w350:refnum<class "ECHARPE_Channel.lvclass">)  [unwired: 7 in]
          n152 = Format Into String(format string="This was the cycle %d out of %d", w336, w339) -> (resulting string=w343:string)  [unwired: 2 in, 1 out]
          n153 = call-dynamic "Send status.vi"("error in (no error)"=w349, "Channel in"=w350) -> ("error out"=w347:errorcluster, "Channel out"=w344:refnum<class "ECHARPE_Channel.lvclass">)  [unwired: 8 in]
          n154 = call "Log debbug message.vi"("error in (no error)"=w347, "String"=w343, "Channel in"=w344) -> ("error out"=w346:errorcluster, "Channel out"=w345:refnum<class "ECHARPE_Channel.lvclass">)  [unwired: 7 in]
        }
        frame "LOG_END_OF_SERIES" {
          n155 = call "write state.vi"("error in (no error)"=w360, "state"="False", "Channel in"=w361) -> ("error out"=w358:errorcluster, "Channel out"=w359:refnum<class "ECHARPE_Channel.lvclass">)  [unwired: 7 in]
          n156 = call "Log info message.vi"("error in (no error)"=w358, "String"="The acquisition of the image series has been finished", "Channel in"=w359) -> ("error out"=w356:errorcluster, "Channel out"=w357:refnum<class "ECHARPE_Channel.lvclass">)  [unwired: 7 in]
        }
        frame "PAUSE_ACQUISITION" {
          n157 = call "Read Acquisition control.vi"("error in (no error)"=w364, "Channel in"=w365) -> ("error out"=w363:errorcluster, "Acquisition control"=w367:T7, "Channel out"=w362:refnum<class "ECHARPE_Channel.lvclass">)  [unwired: 7 in]
          n158 = Unbundle By Name(w367) -> ("Pause acquisition"=w366:bool)
          n159 = Select(t="PAUSE_ACQUISITION", s=w366, f="STOP_ACQUISITION") -> (s? t:f=w368:string)
          n160 = call "write state.vi"("error in (no error)"=w363, "state"=w368, "Channel in"=w362) -> ("error out"=w370:errorcluster, "Channel out"=w369:refnum<class "ECHARPE_Channel.lvclass">)  [unwired: 7 in]
        }
        frame "STOP_ACQUISITION" {
          n161 = call "Read Acquisition control.vi"("error in (no error)"=w391, "Channel in"=w392) -> ("error out"=w390:errorcluster, "Acquisition control"=w389:T7, "Channel out"=w386:refnum<class "ECHARPE_Channel.lvclass">)  [unwired: 7 in]
          n162 = Bundle By Name(cluster=w389, "Stop Acquisition"=FALSE) -> (w388:T7)
          n163 = Unbundle By Name(w389) -> ("Stop Acquisition"=w393:bool)
          n164 = call "Write Acquisition control.vi"("error in (no error)"=w390, "Acquisition control"=w388, "Channel in"=w386) -> ("error out"=w384:errorcluster, "Channel out"=w385:refnum<class "ECHARPE_Channel.lvclass">)  [unwired: 7 in]
          n165 = Select(t="False", s=w393, f="WAIT_EXPOSE_COMMAND") -> (s? t:f=w396:string)
          n166 = call "write state.vi"("error in (no error)"=w384, "state"=w396, "Channel in"=w385) -> ("error out"=w383:errorcluster, "Channel out"=w382:refnum<class "ECHARPE_Channel.lvclass">)  [unwired: 7 in]
          n167 = call-dynamic "Read Classes.vi"("error in (no error)"=w383, "Channel in"=w382) -> ("error out"=w380:errorcluster, "Classes"=w377:T1, "Channel out"=w376:refnum<class "ECHARPE_Channel.lvclass">)  [unwired: 7 in]
          n168 = Not(x=w393) -> (.not. x?=w397:bool)
          n169 = Unbundle By Name(w377) -> ("Sim_CCD.lvclass"=w381:refnum<class "Sim_CCD.lvclass">)
          n170 = Select(t="WAITING_EXPOSE_COMMAND" ("CCD_STATUS"), s=w397, f="IDLE" ("CCD_STATUS")) -> (s? t:f=w400:string)
          n171 = call "Read Camera Status.vi"("error in (no error)"=w380, "CCDCamera in"=w381) -> ("error out"=w402:errorcluster, "camera status"=w404:T6, "CCDCamera out"=w401:refnum<class "Sim_CCD.lvclass">)  [unwired: 7 in]
          n172 = Bundle By Name(cluster=w404, "CCD_STATUS"=w400) -> (w403:T6)
          n173 = call "Write Camera Status.vi"("error in (no error)"=w402, "camera status"=w403, "CCDCamera in"=w401) -> ("error out"=w379:errorcluster, "CCDCamera out"=w375:refnum<class "Sim_CCD.lvclass">)  [unwired: 7 in]
          n174 = Bundle By Name(cluster=w377, "Sim_CCD.lvclass"=w375) -> (w378:T1)
          n175 = call-dynamic "Write Classes.vi"("error in (no error)"=w379, "Classes"=w378, "Channel in"=w376) -> ("error out"=w373:errorcluster, "Channel out"=w374:refnum<class "ECHARPE_Channel.lvclass">)  [unwired: 7 in]
          n176 = case shown="True" w393 {
            tunnel: w374 -> [w408 w413]
            tunnel: [w408 w412] -> w395
            tunnel: [w407 w411] -> w394
            tunnel: w373 -> [w407 w410]
            frame False {
            }
            frame True {
              n177 = call "Log debbug message.vi"("error in (no error)"=w410, "String"="The acquisition has been stopped", "Channel in"=w413) -> ("error out"=w411:errorcluster, "Channel out"=w412:refnum<class "ECHARPE_Channel.lvclass">)  [unwired: 7 in]
            }
          }
        }
        frame "WAIT_EXPOSE_COMMAND" {
          n178 = call "Read Acquisition control.vi"("error in (no error)"=w416, "Channel in"=w417) -> ("error out"=w414:errorcluster, "Acquisition control"=w419:T7, "Channel out"=w415:refnum<class "ECHARPE_Channel.lvclass">)  [unwired: 7 in]
          n179 = Unbundle By Name(w419) -> ("wait expose command"=w418:bool)
          n180 = Select(t="STOP_ACQUISITION", s=w418, f="EXPOSE") -> (s? t:f=w420:string)
          n181 = call "write state.vi"("error in (no error)"=w414, "state"=w420, "Channel in"=w415) -> ("error out"=w422:errorcluster, "Channel out"=w421:refnum<class "ECHARPE_Channel.lvclass">)  [unwired: 7 in]
        }
        frame "------------------------------" {
        }
        frame "SET" {
          n182 = call "Read GUI request.vi"("error in (no error)"=w432, "Channel in"=w431) -> ("error out"=w428:errorcluster, "GUI request"=w430:T2)  [unwired: 7 in, 1 out]
          n183 = Unbundle By Name(w430) -> ("field 2"=w429:string, "field 3"=w427:string)
          n184 = case shown="\"SUFFIX\"" w429 {
            tunnel: [w447 w454 w479 w499 w510 w529 w547] -> w436
            tunnel: w431 -> [w447 w449 w475 w495 w517 w534 w549]
            tunnel: [w446 w453 w478 w498 w509 w528 w546] -> w433
            tunnel: w428 -> [w446 w458 w482 w502 w518 w533 w541]
            tunnel: w427 -> [_ w459 w483 w503 w519 w539 w550]
            frame "False", Default {
            }
            frame "EXPTIME" {
              n185 = call-dynamic "Read Classes.vi"("error in (no error)"=w458, "Channel in"=w449) -> ("error out"=w457:errorcluster, "Classes"=w452:T1, "Channel out"=w448:refnum<class "ECHARPE_Channel.lvclass">)  [unwired: 7 in]
              n186 = Unbundle By Name(w452) -> ("Sim_CCD.lvclass"=w456:refnum<class "Sim_CCD.lvclass">)
              n187 = Fract/Exp String To Number(string=w459, default (0 dbl)=0.0) -> (number=w466:dbl)  [unwired: 2 in, 1 out]
              n188 = call "read new acquisition config.vi"("error in (no error)"=w457, "Simulated_CCD_Camera in"=w456) -> ("error out"=w462:errorcluster, "new acquisition configuration"=w465:T9, "Simulated_CCD_Camera out"=w463:refnum<class "Sim_CCD.lvclass">)  [unwired: 7 in]
              n189 = Bundle By Name(cluster=w465, "EXPTIME"=w466) -> (w464:T9)
              n190 = call "write new acquisition config.vi"("error in (no error)"=w462, "new acquisition configuration"=w464, "Simulated_CCD_Camera in"=w463) -> ("error out"=w461:errorcluster, "Simulated_CCD_Camera out"=w460:refnum<class "Sim_CCD.lvclass">)  [unwired: 7 in]
              n191 = call-dynamic "verify expouse time.vi"("error in (no error)"=w461, "Simulated_CCD_Camera in"=w460) -> ("error out"=w455:errorcluster, "Simulated_CCD_Camera out"=w450:refnum<class "Sim_CCD.lvclass">)  [unwired: 8 in]
              n192 = Bundle By Name(cluster=w452, "Sim_CCD.lvclass"=w450) -> (w451:T1)
              n193 = call-dynamic "Write Classes.vi"("error in (no error)"=w455, "Classes"=w451, "Channel in"=w448) -> ("error out"=w453:errorcluster, "Channel out"=w454:refnum<class "ECHARPE_Channel.lvclass">)  [unwired: 7 in]
            }
            frame "COOLER_POWER_STATUS" {
              n194 = call-dynamic "Read Classes.vi"("error in (no error)"=w482, "Channel in"=w475) -> ("error out"=w481:errorcluster, "Classes"=w477:T1, "Channel out"=w474:refnum<class "ECHARPE_Channel.lvclass">)  [unwired: 7 in]
              n195 = Unbundle By Name(w477) -> ("Sim_CCD.lvclass"=w480:refnum<class "Sim_CCD.lvclass">)
              n196 = Fract/Exp String To Number(string=w483, default (0 dbl)=u16 0) -> (number=w472:u16)  [unwired: 2 in, 1 out]
              n197 = call "read new acquisition config.vi"("error in (no error)"=w481, "Simulated_CCD_Camera in"=w480) -> ("error out"=w484:errorcluster, "new acquisition configuration"=w487:T9, "Simulated_CCD_Camera out"=w485:refnum<class "Sim_CCD.lvclass">)  [unwired: 7 in]
              n198 = Bundle By Name(cluster=w487, "COOLER_POWER_STATUS"=w472) -> (w486:T9)
              n199 = call "write new acquisition config.vi"("error in (no error)"=w484, "new acquisition configuration"=w486, "Simulated_CCD_Camera in"=w485) -> ("error out"=w471:errorcluster, "Simulated_CCD_Camera out"=w470:refnum<class "Sim_CCD.lvclass">)  [unwired: 7 in]
              n200 = call "verify cooler.vi"("error in (no error)"=w471, "Simulated Camera in"=w470) -> ("error out"=w468:errorcluster, "Simulated Camera out"=w469:refnum<class "Sim_CCD.lvclass">)  [unwired: 8 in]
              n201 = Bundle By Name(cluster=w477, "Sim_CCD.lvclass"=w469) -> (w476:T1)
              n202 = call-dynamic "Write Classes.vi"("error in (no error)"=w468, "Classes"=w476, "Channel in"=w474) -> ("error out"=w478:errorcluster, "Channel out"=w479:refnum<class "ECHARPE_Channel.lvclass">)  [unwired: 7 in]
            }
            frame "TEMP" {
              n203 = call-dynamic "Read Classes.vi"("error in (no error)"=w502, "Channel in"=w495) -> ("error out"=w501:errorcluster, "Classes"=w497:T1, "Channel out"=w494:refnum<class "ECHARPE_Channel.lvclass">)  [unwired: 7 in]
              n204 = Unbundle By Name(w497) -> ("Sim_CCD.lvclass"=w500:refnum<class "Sim_CCD.lvclass">)
              n205 = Fract/Exp String To Number(string=w503, default (0 dbl)=0) -> (number=w492:i32)  [unwired: 2 in, 1 out]
              n206 = call "read new acquisition config.vi"("error in (no error)"=w501, "Simulated_CCD_Camera in"=w500) -> ("error out"=w504:errorcluster, "new acquisition configuration"=w507:T9, "Simulated_CCD_Camera out"=w505:refnum<class "Sim_CCD.lvclass">)  [unwired: 7 in]
              n207 = Bundle By Name(cluster=w507, "TEMP"=w492) -> (w506:T9)
              n208 = call "write new acquisition config.vi"("error in (no error)"=w504, "new acquisition configuration"=w506, "Simulated_CCD_Camera in"=w505) -> ("error out"=w491:errorcluster, "Simulated_CCD_Camera out"=w490:refnum<class "Sim_CCD.lvclass">)  [unwired: 7 in]
              n209 = call "verify temperature.vi"("error in (no error)"=w491, "Simulated Camera in"=w490) -> ("error out"=w488:errorcluster, "Simulated Camera out"=w489:refnum<class "Sim_CCD.lvclass">)  [unwired: 8 in]
              n210 = Bundle By Name(cluster=w497, "Sim_CCD.lvclass"=w489) -> (w496:T1)
              n211 = call-dynamic "Write Classes.vi"("error in (no error)"=w488, "Classes"=w496, "Channel in"=w494) -> ("error out"=w498:errorcluster, "Channel out"=w499:refnum<class "ECHARPE_Channel.lvclass">)  [unwired: 7 in]
            }
            frame "#FRAMES" {
              n212 = call-dynamic "Read Classes.vi"("error in (no error)"=w518, "Channel in"=w517) -> ("error out"=w515:errorcluster, "Classes"=w513:T1, "Channel out"=w508:refnum<class "ECHARPE_Channel.lvclass">)  [unwired: 7 in]
              n213 = Unbundle By Name(w513) -> ("Sim_CCD.lvclass"=w516:refnum<class "Sim_CCD.lvclass">)
              n214 = Fract/Exp String To Number(string=w519, default (0 dbl)=u32 0) -> (number=w520:u32)  [unwired: 2 in, 1 out]
              n215 = call "read new acquisition config.vi"("error in (no error)"=w515, "Simulated_CCD_Camera in"=w516) -> ("error out"=w523:errorcluster, "new acquisition configuration"=w526:T9, "Simulated_CCD_Camera out"=w524:refnum<class "Sim_CCD.lvclass">)  [unwired: 7 in]
              n216 = Bundle By Name(cluster=w526, "#FRAMES"=w520) -> (w525:T9)
              n217 = call "write new acquisition config.vi"("error in (no error)"=w523, "new acquisition configuration"=w525, "Simulated_CCD_Camera in"=w524) -> ("error out"=w521:errorcluster, "Simulated_CCD_Camera out"=w522:refnum<class "Sim_CCD.lvclass">)  [unwired: 7 in]
              n218 = call "verify #frames.vi"("error in (no error)"=w521, "Simulated_CCD_Camera in"=w522) -> ("error out"=w514:errorcluster, "Simulated_CCD_Camera out"=w512:refnum<class "Sim_CCD.lvclass">)  [unwired: 8 in]
              n219 = Bundle By Name(cluster=w513, "Sim_CCD.lvclass"=w512) -> (w511:T1)
              n220 = call-dynamic "Write Classes.vi"("error in (no error)"=w514, "Classes"=w511, "Channel in"=w508) -> ("error out"=w509:errorcluster, "Channel out"=w510:refnum<class "ECHARPE_Channel.lvclass">)  [unwired: 7 in]
            }
            frame "#CYCLES" {
              n221 = Fract/Exp String To Number(string=w539, default (0 dbl)=u32 0) -> (number=w537:u32)  [unwired: 2 in, 1 out]
              n222 = call-dynamic "read new acq config.vi"("error in (no error)"=w533, "Channel in"=w534) -> ("error out"=w536:errorcluster, "new acq config"=w538:cluster{"suffix":string, "#CYCLES":u32}, "Channel out"=w535:refnum<class "ECHARPE_Channel.lvclass">)  [unwired: 7 in]
              n223 = Bundle By Name(cluster=w538, "#CYCLES"=w537) -> (w532:cluster{"suffix":string, "#CYCLES":u32})
              n224 = call-dynamic "Write new acq config.vi"("error in (no error)"=w536, "new acq config"=w532, "Channel in"=w535) -> ("error out"=w531:errorcluster, "Channel out"=w530:refnum<class "ECHARPE_Channel.lvclass">)  [unwired: 7 in]
              n225 = call "verify #cycles.vi"("error in (no error)"=w531, "Channel in"=w530) -> ("error out"=w528:errorcluster, "Channel out"=w529:refnum<class "ECHARPE_Channel.lvclass">)  [unwired: 8 in]
            }
            frame "SUFFIX" {
              n226 = To Lower Case(string=w550) -> (all lower case string=w543:string)
              n227 = call-dynamic "read new acq config.vi"("error in (no error)"=w541, "Channel in"=w549) -> ("error out"=w545:errorcluster, "new acq config"=w544:cluster{"suffix":string, "#CYCLES":u32}, "Channel out"=w548:refnum<class "ECHARPE_Channel.lvclass">)  [unwired: 7 in]
              n228 = Bundle By Name(cluster=w544, "suffix"=w543) -> (w542:cluster{"suffix":string, "#CYCLES":u32})
              n229 = call-dynamic "Write new acq config.vi"("error in (no error)"=w545, "new acq config"=w542, "Channel in"=w548) -> ("error out"=w546:errorcluster, "Channel out"=w547:refnum<class "ECHARPE_Channel.lvclass">)  [unwired: 7 in]
            }
          }
          n230 = call-dynamic "update camera op mode error.vi"("error in (no error)"=w433, "Channel in"=w436) -> ("error out"=w437:errorcluster, "Channel out"=w438:refnum<class "ECHARPE_Channel.lvclass">)  [unwired: 8 in]
          n231 = call-dynamic "log acq config errors.vi"("error in (no error)"=w437, "Channel in"=w438) -> ("error out"=w434:errorcluster, "Channel out"=w435:refnum<class "ECHARPE_Channel.lvclass">)  [unwired: 8 in]
          n232 = call "write acquisition config.vi"("error in (no error)"=w434, "Channel in"=w435) -> ("error out"=w440:errorcluster, "Channel out"=w439:refnum<class "ECHARPE_Channel.lvclass">)  [unwired: 8 in]
          n233 = call-dynamic "Send status.vi"("error in (no error)"=w440, "Channel in"=w439) -> ("error out"=w444:errorcluster, "Channel out"=w445:refnum<class "ECHARPE_Channel.lvclass">)  [unwired: 8 in]
          n234 = call "write state.vi"("error in (no error)"=w444, "state"="False", "Channel in"=w445) -> ("error out"=w442:errorcluster, "Channel out"=w443:refnum<class "ECHARPE_Channel.lvclass">)  [unwired: 7 in]
        }
      }
    }
    frame Error {
    }
  }
  "error out" <- w3
  "Channel out" <- w1
